vi "test.vi"() -> ()   [LabVIEW 2012]
uses:
  Program Files/CAEN/HV/CAENHVWrapper/labview/CAENHVWrapper/CAENHVWrapper.lvlib
panel:
  in  "HV Cluster":T1={"HV Power On/Off"=[], "Set Voltage"=[], "HV Tolerance (%)"=1.0}
  out "error out":errorcluster
  in  "error in":errorcluster
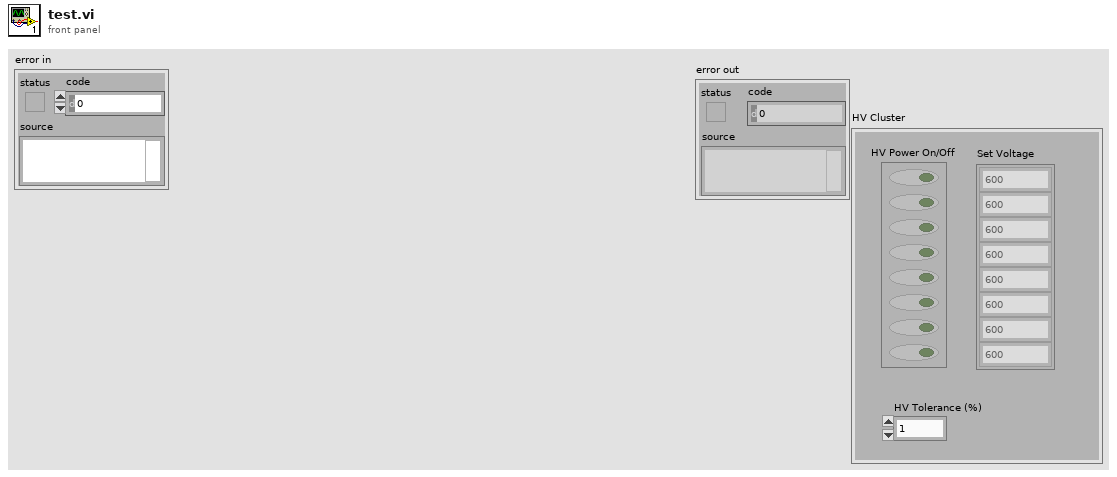
[diagram p1: front panel]
types:
  T1 = cluster{"HV Power On/Off":bool[], "Set Voltage":string[], "HV Tolerance (%)":dbl}
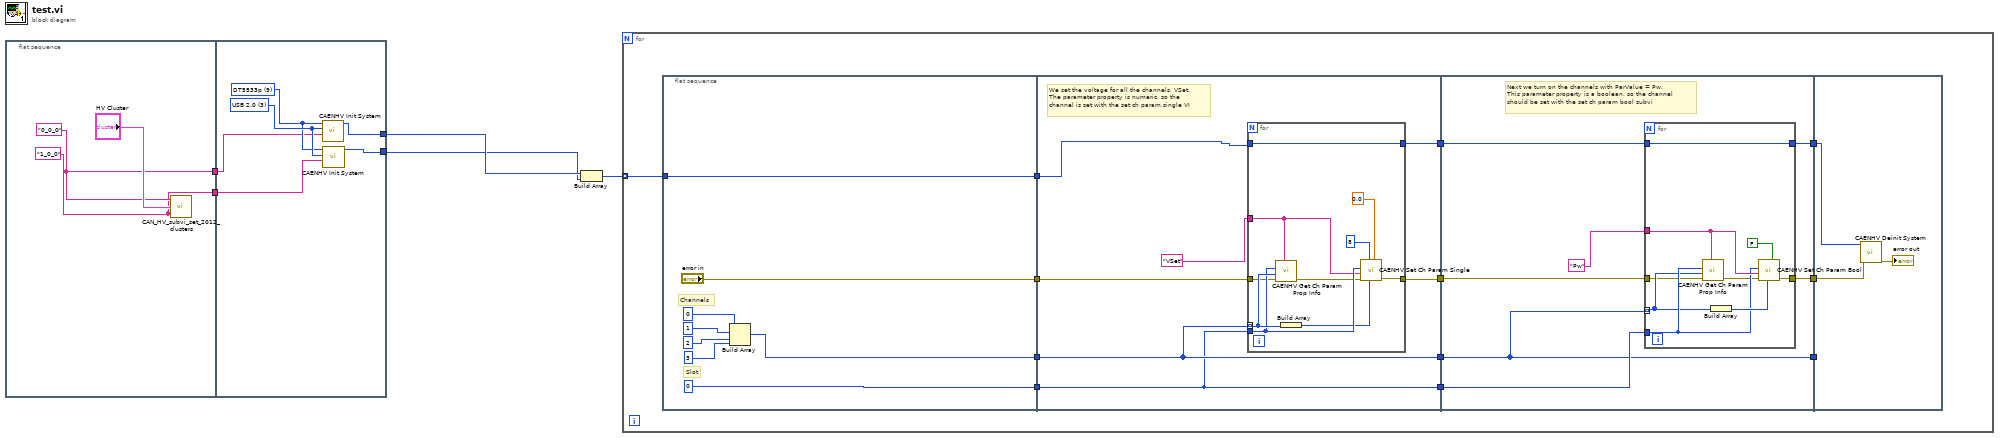
[diagram p0: block diagram]
diagram:
  n1 = flat-sequence {
    tunnel: [w7] -> w4
    tunnel: [w6] -> w3
    tunnel: w4 -> [w12]
    tunnel: w3 -> [w11]
    tunnel: [w10] -> w2
    tunnel: [w9] -> w1
    frame #0 {
      w6 = "1_0_0"
      w7 = "0_0_0"
      n2 = call "CAN_HV_subvi_set_2012_clusters.vi"("IP adress HV2"=w6, "HV Cluster"="HV Cluster", "IP adress HV1"=w7) -> ()  [unwired: 2 out]
    }
    frame #1 {
      w14 = 3 items=["TCP/IP"=0, "HS CAENET"=2, "USB 2.0"=3, "CONET Optical Link"=4, "USB VCP"=5] ("LinkType")
      w13 = u32 9 items=["SY1527", "SY2527", "SY4527", "SY5527", "N568", "V65XX", "N1470", "V8100", "", "DT5533p"] ("system")
      n3 = call "CAENHV Init System.vi"("Arg"=w12, "LinkType"=w14, "system"=w13) -> ("handle"=w10:i32)  [unwired: 7 in, 1 out]
      n4 = call "CAENHV Init System.vi"("Arg"=w11, "LinkType"=w14, "system"=w13) -> ("handle"=w9:i32)  [unwired: 7 in, 1 out]
    }
  }
  n5 = Build Array(w2, w1) -> (w5:i32[])
  n6 = for {
    tunnel: w5 -> [w15] mode=indexing
    n7 = flat-sequence {
      tunnel: [w34] -> w26
      tunnel: [0] -> w25
      tunnel: ["error in"] -> w24
      tunnel: [w27] -> w16
      tunnel: w15 -> [w27]
      tunnel: [w41] -> w23
      tunnel: [w38] -> w22
      tunnel: [w40] -> w21
      tunnel: [w39] -> w20
      tunnel: w26 -> [w39]
      tunnel: w25 -> [w38]
      tunnel: w24 -> [w36]
      tunnel: w16 -> [w35]
      tunnel: w23 -> [w57]
      tunnel: w22 -> [w53]
      tunnel: w21 -> [w56]
      tunnel: w20 -> [w52]
      tunnel: [w55] -> w19
      tunnel: [w54] -> w18
      tunnel: [w52] -> w17
      tunnel: w19 -> [w68]
      tunnel: w18 -> [w69]
      tunnel: w17 -> [_]
      frame #0 {
        # "Slot"
        # "Channels"
        n8 = Build Array(0, 1, 2, 3) -> (w34:i32[])
      }
      frame #1 {
        # "We set the voltage for all the channels, VSet.\nThe parameter property is numeric, so the\nchannel is set with the set ch param single VI"
        n9 = for {
          tunnel: "VSet" ("Setvoltage") -> [w49]
          tunnel: w39 -> [w51] mode=indexing
          tunnel: w38 -> [w50]
          tunnel: w35 -> [w42]
          tunnel: [w42] -> w41
          tunnel: [w48] -> w40
          tunnel: w36 -> [w43]
          n10 = call "CAENHV Get Ch Param Prop Info.vi"("ParName"=w49, "error in (no error)"=w43, "Ch"=w51, "slot"=w50) -> ("error out"=w46:errorcluster)  [unwired: 5 in, 2 out]
          n11 = Build Array(w51) -> (w47:i32[])
          n12 = call "CAENHV Set Ch Param Single.vi"("ParValue"=sgl 0.0, "ChList"=w47, "ChNum (1)"=u16 8, "error in (no error)"=w46, "ParName"=w49, "slot"=w50) -> ("error out"=w48:errorcluster)  [unwired: 5 in]
        }
      }
      frame #2 {
        # "Next we turn on the channels with ParValue = Pw. \nThis parameter property is a boolean, so the channel\nshould be set with the set ch param bool subvi"
        n13 = for {
          tunnel: [w67] -> w54
          tunnel: "Pw" ("ParName") -> [w66]
          tunnel: w57 -> [w59]
          tunnel: [w59] -> w55
          tunnel: w53 -> [w64]
          tunnel: w52 -> [w63] mode=indexing
          tunnel: w56 -> [w62]
          n14 = call "CAENHV Get Ch Param Prop Info.vi"("ParName"=w66, "error in (no error)"=w62, "Ch"=w63, "slot"=w64) -> ("error out"=w61:errorcluster)  [unwired: 5 in, 2 out]
          n15 = Build Array(w63) -> (w65:i32[])
          n16 = call "CAENHV Set Ch Param Bool.vi"("ParValue"=FALSE, "ChList"=w65, "error in (no error)"=w61, "ParName"=w66, "slot"=w64) -> ("error out"=w67:errorcluster)  [unwired: 6 in]
        }
      }
      frame #3 {
        n17 = call "CAENHV Deinit System.vi"("error in (no error)"=w69, "handle"=w68) -> ("error out"=→"error out":errorcluster)  [unwired: 9 in]
      }
    }
  }
